vi "Rabi Pulse 4.vi"() -> ()   [LabVIEW 2012]
uses:
  <vilib>/DAQmx/read.llb/DAQmx Read (Digital Bool 1Line 1Point).vi
  <vilib>/DAQmx/create/channels.llb/DAQmx Create Channel (DI-Digital Input).vi
  <vilib>/Utility/file.llb/Write To Spreadsheet File (DBL).vi
  <vilib>/DAQmx/miscellaneous.llb/DAQmx Fill In Error Info.vi
panel:
  in  "read out trigger length":dbl
  in  "N Loop":i32=25000
  in  "AOM read out length":dbl
  out "Run":bool
  out "size(s)":i32=225
  in  "file path (dialog if empty)":path=path "C:/Users/Ouyang Group/Documents/Data/12-5-13/Rabi pulse sequence 7"
  in  "AOM Init length":dbl=3e-07
  in  "Path to spinapi.dll":path=path "C:/SpinCore/SpinAPI/dll/spinapi64.dll"
  in  "stop":bool
  in  "start/restart":bool
  in  "MW width Max":dbl=5e-07
  in  "MW width step size":dbl=2e-09
  in  "MW width Min":dbl=5e-08
  in  "clock_freq (MHz)":dbl=300.0
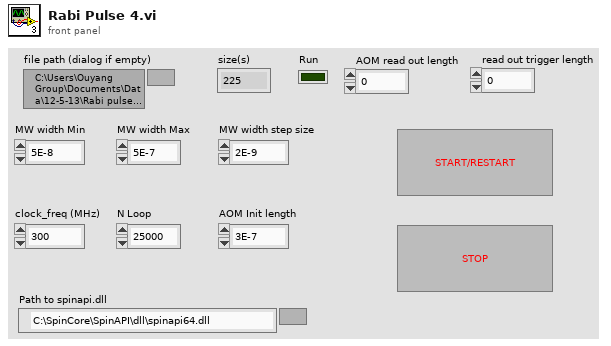
[diagram p1: front panel]
types:
  T1 = cluster{"Instruct Data":i32, "Op Code":i32, "Flags":bool[], "Comments":string, "Time (s)":dbl}[]
  T2 = cluster{"Instruct Data":i32, "Op Code":i32, "Flags":bool[], "Comments":string, "Time (s)":dbl}
  T3 = enum16{"Pulse Program", "Frequency Registers", "TX Phase Registers", "RX Phase Registers"}
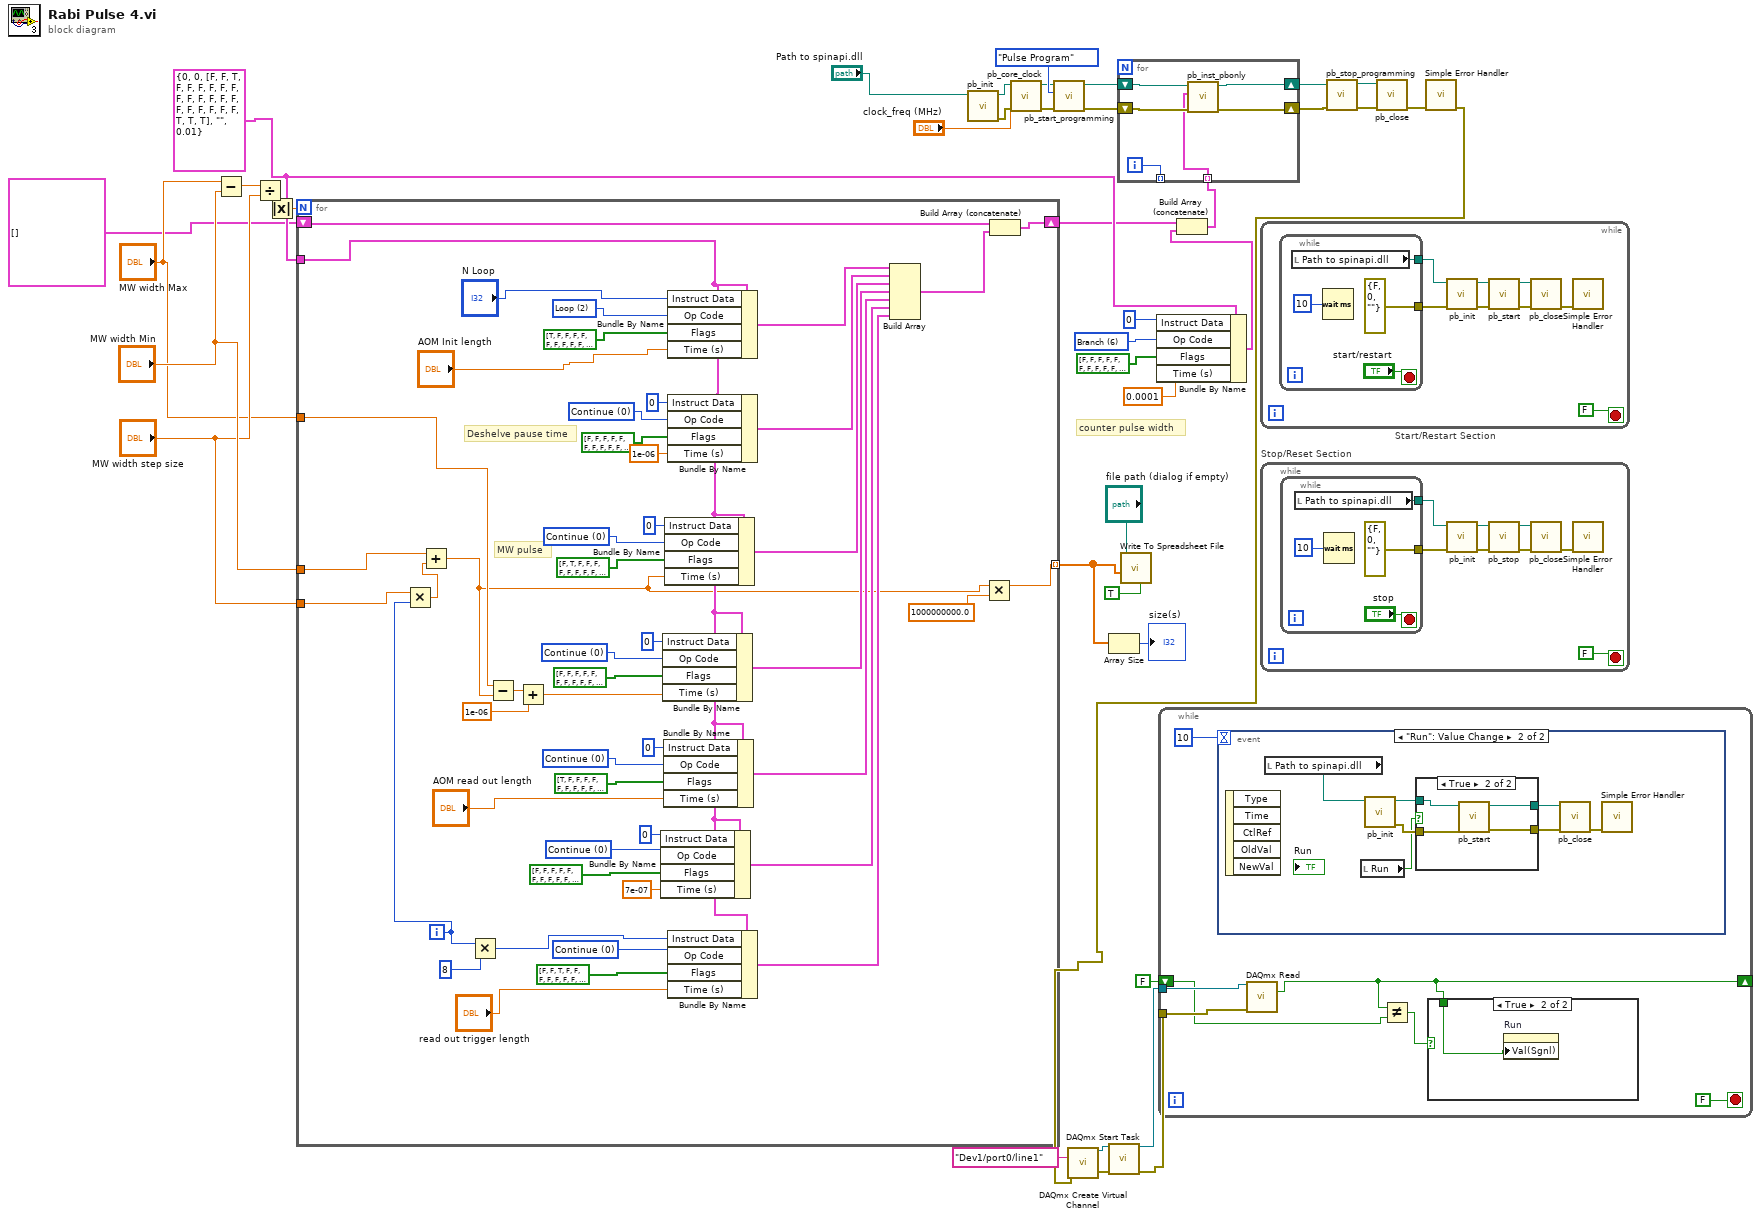
[diagram p0: block diagram]
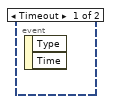
[diagram p2: hidden frame]
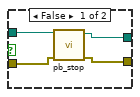
[diagram p3: hidden frame]
diagram:
  w7 = 6 items=["Continue", "Stop", "Loop", "End Loop", "JSR", "RTS", "Branch", "Long Delay", "Wait"] ("Op Code")
  w5 = T2 {"Instruct Data"=0, "Op Code"=0, "Flags"=[FALSE, FALSE, TRUE, FALSE, FALSE, FALSE, FALSE, FALSE, FALSE, FALSE, FALSE, FALSE, FALSE, FALSE, FALSE, FALSE, FALSE, FALSE, FALSE, FALSE, FALSE, TRUE, TRUE, TRUE], "Comments"="", "Time (s)"=0.01} ("PB Inst 2")
  # "counter pulse width"
  n1 = Subtract(x="MW width Max", y="MW width Min") -> (x-y=w28:dbl)
  n2 = Divide(x=w28, y="MW width step size") -> (x/y=w27:dbl)
  n3 = Absolute Value(x=w27) -> (abs(x)=w10:dbl)
  n4 = for {
    N: w10 -> [_]
    tunnel: "MW width Min" -> [w52]
    tunnel: "MW width step size" -> [w53]
    tunnel: [w77] -> w20 mode=indexing
    tunnel: w5 -> [w66]
    shift-right: [w88] -> w3
    shift-left: T1 [] -> [w89]
    tunnel: "MW width Max" -> [w49]
    i -> [w54]
    w57 = 0 items=["Continue", "Stop", "Loop", "End Loop", "JSR", "RTS", "Branch", "Long Delay", "Wait"] ("Op Code")
    w60 = 2 items=["Continue", "Stop", "Loop", "End Loop", "JSR", "RTS", "Branch", "Long Delay", "Wait"] ("Op Code")
    w68 = 0 items=["Continue", "Stop", "Loop", "End Loop", "JSR", "RTS", "Branch", "Long Delay", "Wait"] ("Op Code")
    w71 = 0 items=["Continue", "Stop", "Loop", "End Loop", "JSR", "RTS", "Branch", "Long Delay", "Wait"] ("Op Code")
    w75 = 0 items=["Continue", "Stop", "Loop", "End Loop", "JSR", "RTS", "Branch", "Long Delay", "Wait"] ("Op Code")
    w83 = 0 items=["Continue", "Stop", "Loop", "End Loop", "JSR", "RTS", "Branch", "Long Delay", "Wait"] ("Op Code")
    w86 = 0 items=["Continue", "Stop", "Loop", "End Loop", "JSR", "RTS", "Branch", "Long Delay", "Wait"] ("Op Code")
    # "MW pulse"
    # "Deshelve pause time"
    n5 = Multiply(x=w53, y=w54) -> (x*y=w55:dbl)
    n6 = Add(x=w52, y=w55) -> (x+y=w48:dbl)
    n7 = Multiply(x=w54, y=8) -> (x*y=w44:i32)
    n8 = Subtract(x=w49, y=w48) -> (x-y=w47:dbl)
    n9 = Add(x=w47, y=1e-06) -> (x+y=w45:dbl)
    n10 = Bundle By Name(cluster=w66, "Instruct Data"=0, "Op Code"=w75, "Flags"=bool[] [FALSE, FALSE, FALSE, FALSE, FALSE, FALSE, FALSE, FALSE, FALSE, FALSE, FALSE, FALSE, FALSE, FALSE, FALSE, FALSE, FALSE, FALSE, FALSE, FALSE, FALSE, TRUE, TRUE, TRUE], "Time (s)"=7e-07) -> (w62:T2)
    n11 = Bundle By Name(cluster=w66, "Instruct Data"=0, "Op Code"=w68, "Flags"=bool[] [FALSE, FALSE, FALSE, FALSE, FALSE, FALSE, FALSE, FALSE, FALSE, FALSE, FALSE, FALSE, FALSE, FALSE, FALSE, FALSE, FALSE, FALSE, FALSE, FALSE, FALSE, TRUE, TRUE, TRUE], "Time (s)"=w45) -> (w64:T2)
    n12 = Bundle By Name(cluster=w66, "Instruct Data"=0, "Op Code"=w83, "Flags"=bool[] [TRUE, FALSE, FALSE, FALSE, FALSE, FALSE, FALSE, FALSE, FALSE, FALSE, FALSE, FALSE, FALSE, FALSE, FALSE, FALSE, FALSE, FALSE, FALSE, FALSE, FALSE, TRUE, TRUE, TRUE], "Time (s)"="AOM read out length") -> (w65:T2)
    n13 = Bundle By Name(cluster=w66, "Instruct Data"=0, "Op Code"=w86, "Flags"=bool[] [FALSE, TRUE, FALSE, FALSE, FALSE, FALSE, FALSE, FALSE, FALSE, FALSE, FALSE, FALSE, FALSE, FALSE, FALSE, FALSE, FALSE, FALSE, FALSE, FALSE, FALSE, TRUE, TRUE, TRUE], "Time (s)"=w48) -> (w80:T2)
    n14 = Bundle By Name(cluster=w66, "Instruct Data"="N Loop", "Op Code"=w60, "Flags"=bool[] [TRUE, FALSE, FALSE, FALSE, FALSE, FALSE, FALSE, FALSE, FALSE, FALSE, FALSE, FALSE, FALSE, FALSE, FALSE, FALSE, FALSE, FALSE, FALSE, FALSE, FALSE, TRUE, TRUE, TRUE], "Time (s)"="AOM Init length") -> (w82:T2)
    n15 = Bundle By Name(cluster=w66, "Instruct Data"=0, "Op Code"=w57, "Flags"=bool[] [FALSE, FALSE, FALSE, FALSE, FALSE, FALSE, FALSE, FALSE, FALSE, FALSE, FALSE, FALSE, FALSE, FALSE, FALSE, FALSE, FALSE, FALSE, FALSE, FALSE, FALSE, TRUE, TRUE, TRUE], "Time (s)"=1e-06) -> (w81:T2)
    n16 = Bundle By Name(cluster=w66, "Instruct Data"=w44, "Op Code"=w71, "Flags"=bool[] [FALSE, FALSE, TRUE, FALSE, FALSE, FALSE, FALSE, FALSE, FALSE, FALSE, FALSE, FALSE, FALSE, FALSE, FALSE, FALSE, FALSE, FALSE, FALSE, FALSE, FALSE, TRUE, TRUE, TRUE], "Time (s)"="read out trigger length") -> (w63:T2)
    n17 = Build Array(w82, w81, w80, w64, w65, w62, w63) -> (w78:T1)
    n18 = Multiply(x=w48, y=1000000000.0) -> (x*y=w77:dbl)
    n19 = Build Array (concatenate)(w89, w78) -> (w88:T1)
  }
  n20 = call "pb_init.vi"("path in"="Path to spinapi.dll") -> ("error out"=w35:errorcluster, "path out"=w37:path)  [unwired: 3 in, 6 out]
  n21 = call "pb_core_clock.vi"("error in (no error)"=w35, "clock_freq (MHz)"="clock_freq (MHz)", "path in"=w37) -> ("error out"=w34:errorcluster, "path out"=w36:path)  [unwired: 7 in]
  n22 = call "pb_start_programming.vi"("error in (no error)"=w34, "Device"=T3."Pulse Program", "path in"=w36) -> ("error out"=w31:errorcluster, "path out"=w32:path)  [unwired: 1 in, 6 out]
  n23 = Array Size(array=w20) -> (size(s)=→"size(s)":i32)
  n24 = call-poly <vilib>:"Write To Spreadsheet File.vi"("transpose? (no:F)"=TRUE, "1D data"=w20, "file path (dialog if empty)"="file path (dialog if empty)") -> ()  [unwired: 5 in, 1 out]
  n25 = Bundle By Name(cluster=w5, "Instruct Data"=0, "Op Code"=w7, "Flags"=bool[] [FALSE, FALSE, FALSE, FALSE, FALSE, FALSE, FALSE, FALSE, FALSE, FALSE, FALSE, FALSE, FALSE, FALSE, FALSE, FALSE, FALSE, FALSE, FALSE, FALSE, FALSE, TRUE, TRUE, TRUE], "Time (s)"=0.0001) -> (w4:T2)
  n26 = Build Array (concatenate)(w3, w4) -> (w2:T1)
  n27 = for {
    shift-right: [w93] -> w30
    shift-left: w32 -> [w95]
    shift-right: [w92] -> w29
    shift-left: w31 -> [w94]
    tunnel: [w91] -> _ mode=indexing
    tunnel: w2 -> [w90] mode=indexing
    i -> [w91]
    n28 = call "pb_inst_pbonly.vi"("error in (no error)"=w94, "PB Instruction"=w90, "path in"=w95) -> ("error out"=w92:errorcluster, "path out"=w93:path)  [unwired: 2 in, 5 out]
  }
  n29 = while "Start/Restart Section" {
    stop <- FALSE stop-if-true
    n30 = while {
      tunnel: [errorcluster {"status"=FALSE, "code"=0, "source"=""} ("error in (no error)")] -> w100
      tunnel: [w104] -> w96
      stop <- "start/restart" stop-if-true
      n31 = local read "Path to spinapi.dll"() -> (w104:path)
      n32 = Wait (ms)(milliseconds to wait=u32 10) -> ()  [unwired: 1 out]
    }
    n33 = call "pb_init.vi"("error in (no error)"=w100, "path in"=w96) -> ("error out"=w99:errorcluster, "path out"=w102:path)  [unwired: 1 in, 7 out]
    n34 = call "pb_start.vi"("error in (no error)"=w99, "path in"=w102) -> ("error out"=w98:errorcluster, "path out"=w103:path)  [unwired: 1 in, 7 out]
    n35 = call "pb_close.vi"("error in (no error)"=w98, "path in"=w103) -> ("error out"=w97:errorcluster)  [unwired: 9 out]
    n36 = call <vilib>:"Simple Error Handler.vi"("error in (no error)"=w97) -> ()  [unwired: 1 in, 8 out]
  }
  n37 = while "Stop/Reset Section" {
    stop <- FALSE stop-if-true
    n38 = while {
      tunnel: [errorcluster {"status"=FALSE, "code"=0, "source"=""} ("error in (no error)")] -> w112
      tunnel: [w116] -> w108
      stop <- "stop" stop-if-true
      n39 = local read "Path to spinapi.dll"() -> (w116:path)
      n40 = Wait (ms)(milliseconds to wait=u32 10) -> ()  [unwired: 1 out]
    }
    n41 = call "pb_init.vi"("error in (no error)"=w112, "path in"=w108) -> ("error out"=w111:errorcluster, "path out"=w114:path)  [unwired: 1 in, 7 out]
    n42 = call "pb_stop.vi"("error in (no error)"=w111, "path in"=w114) -> ("error out"=w110:errorcluster, "path out"=w115:path)  [unwired: 8 out]
    n43 = call "pb_close.vi"("error in (no error)"=w110, "path in"=w115) -> ("error out"=w109:errorcluster)  [unwired: 9 out]
    n44 = call <vilib>:"Simple Error Handler.vi"("error in (no error)"=w109) -> ()  [unwired: 1 in, 8 out]
  }
  n45 = call "pb_stop_programming.vi"("error in (no error)"=w29, "path in"=w30) -> ("error out"=w38:errorcluster, "path out"=w39:path)  [unwired: 1 in, 7 out]
  n46 = call "pb_close.vi"("error in (no error)"=w38, "path in"=w39) -> ("error out"=w23:errorcluster)  [unwired: 9 out]
  n47 = call <vilib>:"Simple Error Handler.vi"("error in (no error)"=w23) -> ("error out"=w14:errorcluster)  [unwired: 1 in, 7 out]
  n48 = call-poly <vilib>:"DAQmx Create Virtual Channel.vi"("lines"=tag "Dev1/port0/line1", "error in"=w14) -> ("task out"=w12:refnum<k21>, "error out"=w11:errorcluster)  [unwired: 12 in]
  n49 = call <vilib>:"DAQmx Start Task.vi"("task/channels in"=w12, "error in"=w11) -> ("task out"=w13:refnum<k21>, "error out"=w16:errorcluster)  [unwired: 12 in]
  n50 = while {
    tunnel: w13 -> [w126]
    tunnel: w16 -> [w125]
    shift-right: [w122] -> _
    shift-left: FALSE ("data") -> [w124]
    stop <- FALSE stop-if-true
    n51 = event shown="[1] \"Run\": Value Change" {
      selector: _ -> [_ _]
      dyn-events: _ -> [_ _]
      timeout: 10 -> [_ _]
      event Timeout {
        n52 = event-data() -> ()  [unwired: 1 in, 2 out]
      }
      event "Run": Value Change {
        n53 = event-data() -> ()  [unwired: 1 in, 5 out]
        n54 = local read "Path to spinapi.dll"() -> (w127:path)
        n55 = local read "Run"() -> (w131:bool)
        n56 = call "pb_init.vi"("path in"=w127) -> ("error out"=w132:errorcluster, "path out"=w133:path)  [unwired: 2 in, 7 out]
        n57 = case shown="True" w131 {
          tunnel: w133 -> [w137 w141]
          tunnel: w132 -> [w136 w140]
          tunnel: [w135 w139] -> w129
          tunnel: [w134 w138] -> w128
          frame False {
            n58 = call "pb_stop.vi"("error in (no error)"=w136, "path in"=w137) -> ("error out"=w134:errorcluster, "path out"=w135:path)  [unwired: 8 out]
          }
          frame True {
            n59 = call "pb_start.vi"("error in (no error)"=w140, "path in"=w141) -> ("error out"=w138:errorcluster, "path out"=w139:path)  [unwired: 1 in, 7 out]
          }
        }
        n60 = call "pb_close.vi"("error in (no error)"=w128, "path in"=w129) -> ("error out"=w130:errorcluster)  [unwired: 9 out]
        n61 = call <vilib>:"Simple Error Handler.vi"("error in (no error)"=w130) -> ()  [unwired: 1 in, 8 out]
      }
    }
    n62 = call-poly <vilib>:"DAQmx Read.vi"("task/channels in"=w126, "error in"=w125) -> ("data"=w122:bool)  [unwired: 11 in, 2 out]
    n63 = Not Equal?(x=w122, y=w124) -> (x != y?=w123:bool)
    n64 = case shown="True" w123 {
      tunnel: w122 -> [_ w142]
      frame False {
      }
      frame True {
        n65 = property on="Run" class="Bool (strict)"("Val(Sgnl)"=w142) -> ()  [unwired: 2 in, 2 out]
      }
    }
  }
